vi "TCS_VISA.vi"() -> ()   [LabVIEW 2018]
uses:
  RxTx/RxTx.lvclass
  Serial Communication/Serial Communication.lvclass
  Serial Communication/Serial Communication.lvclass/Serial Communication.ctl
panel:
  in  "RxTx.lvclass 2":refnum<class "RxTx.lvclass">
  in  "Serial Communication in":refnum<class "Serial Communication.lvclass">
  in  "RxTx.lvclass":refnum<class "RxTx.lvclass">
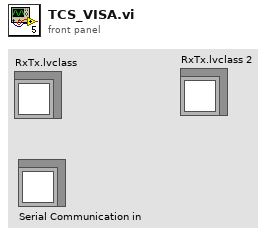
[diagram p1: front panel]
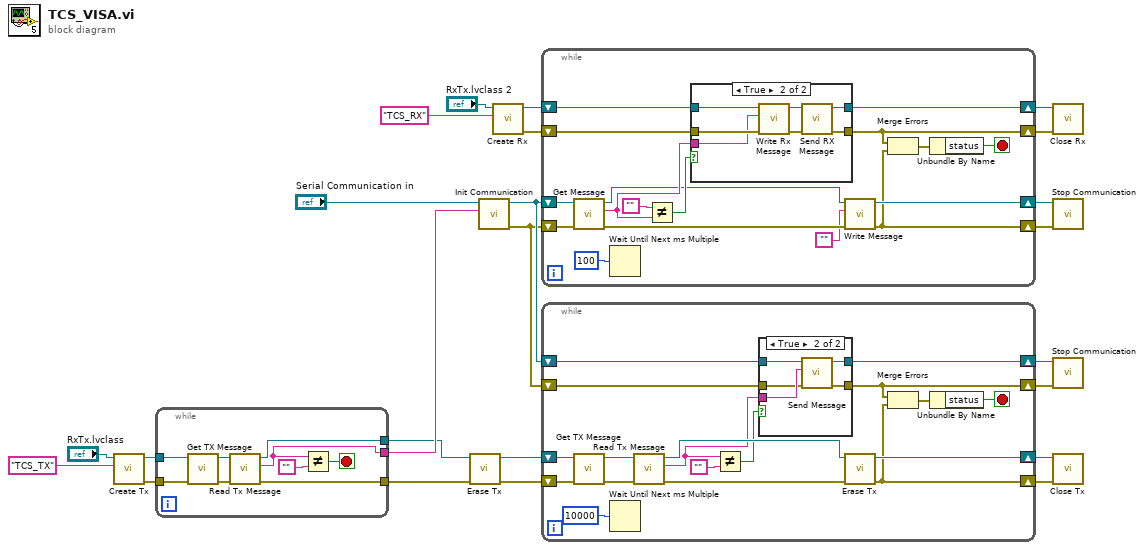
[diagram p0: block diagram]
diagram:
  n1 = call "Create Tx.vi"("Writer Name"="TCS_TX" ("Reader Name"), "RxTx in"="RxTx.lvclass") -> ("error out"=w8:errorcluster, "RxTx out"=w9:refnum<class "RxTx.lvclass">)  [unwired: 8 in]
  n2 = while {
    tunnel: w9 -> [w30]
    tunnel: w8 -> [w29]
    tunnel: [w28] -> w2
    tunnel: [w27] -> w1
    tunnel: [w25] -> w7
    stop <- w26 stop-if-true
    n3 = call "Get TX Message.vi"("error in (no error)"=w29, "RxTx in"=w30) -> ("error out"=w33:errorcluster, "RxTx out"=w32:refnum<class "RxTx.lvclass">)  [unwired: 8 in]
    n4 = call "Read Tx Message.vi"("error in (no error)"=w33, "RxTx in"=w32) -> ("error out"=w28:errorcluster, "Tx Message"=w25:string, "RxTx out"=w27:refnum<class "RxTx.lvclass">)  [unwired: 7 in]
    n5 = Not Equal?(x=w25, y="") -> (x != y?=w26:bool)
  }
  n6 = call "Erase Tx.vi"("error in (no error)"=w2, "RxTx in"=w1) -> ("error out"=w4:errorcluster, "RxTx out"=w3:refnum<class "RxTx.lvclass">)  [unwired: 8 in]
  n7 = call "Init Communication.vi"("VISA resource name"=w7, "Serial Communication in"="Serial Communication in") -> ("error out"=w5:errorcluster, "Serial Communication out"=w6:refnum<class "Serial Communication.lvclass">)  [unwired: 8 in]
  n8 = call "Create Rx.vi"("Reader Name"="TCS_RX", "RxTx in"="RxTx.lvclass 2") -> ("error out"=w14:errorcluster, "RxTx out"=w15:refnum<class "RxTx.lvclass">)  [unwired: 8 in]
  n9 = while {
    shift-right: [w36] -> w10
    shift-left: w5 -> [w43]
    shift-right: [w37] -> w11
    shift-left: w6 -> [w42]
    shift-right: [w46] -> w12
    shift-left: w14 -> [w50]
    shift-right: [w48] -> w13
    shift-left: w15 -> [w49]
    stop <- w34 stop-if-true
    n10 = call "Get Message.vi"("error in (no error)"=w43, "Serial Communication in"=w42) -> ("error out"=w39:errorcluster, "Message"=w41:string, "Serial Communication out"=w40:refnum<class "Serial Communication.lvclass">)  [unwired: 7 in]
    n11 = Wait Until Next ms Multiple(millisecond multiple=u32 100 ("milliseconds to wait")) -> ()  [unwired: 1 out]
    n12 = Not Equal?(x="", y=w41) -> (x != y?=w44:bool)
    n13 = case shown="True" w44 {
      tunnel: w50 -> [w51 w57]
      tunnel: w49 -> [w52 w56]
      tunnel: w41 -> [_ w55]
      tunnel: [w52 w54] -> w48
      tunnel: [w51 w53] -> w46
      frame False {
      }
      frame True {
        n14 = call "Write Rx Message.vi"("error in (no error)"=w57, "Rx Message"=w55, "RxTx in"=w56) -> ("error out"=w58:errorcluster, "RxTx out"=w59:refnum<class "RxTx.lvclass">)  [unwired: 7 in]
        n15 = call "Send RX Message.vi"("error in (no error)"=w58, "RxTx in"=w59) -> ("error out"=w53:errorcluster, "RxTx out"=w54:refnum<class "RxTx.lvclass">)  [unwired: 8 in]
      }
    }
    n16 = call "Write Message.vi"("error in (no error)"=w39, "Message"="", "Serial Communication in"=w40) -> ("error out"=w36:errorcluster, "Serial Communication out"=w37:refnum<class "Serial Communication.lvclass">)  [unwired: 7 in]
    n17 = Merge Errors(w46, w36) -> (w47:errorcluster)
    n18 = Unbundle By Name(w47) -> ("status"=w34:bool)
  }
  n19 = while {
    shift-right: [w69] -> w19
    shift-left: w5 -> [w71]
    shift-right: [w70] -> w20
    shift-left: w6 -> [w72]
    shift-right: [w64] -> w22
    shift-left: w4 -> [w73]
    shift-right: [w66] -> w23
    shift-left: w3 -> [w74]
    stop <- w60 stop-if-true
    n20 = call "Get TX Message.vi"("error in (no error)"=w73, "RxTx in"=w74) -> ("error out"=w76:errorcluster, "RxTx out"=w75:refnum<class "RxTx.lvclass">)  [unwired: 8 in]
    n21 = Wait Until Next ms Multiple(millisecond multiple=u32 10000 ("milliseconds to wait")) -> ()  [unwired: 1 out]
    n22 = call "Read Tx Message.vi"("error in (no error)"=w76, "RxTx in"=w75) -> ("error out"=w65:errorcluster, "Tx Message"=w61:string, "RxTx out"=w67:refnum<class "RxTx.lvclass">)  [unwired: 7 in]
    n23 = Not Equal?(x=w61, y="") -> (x != y?=w63:bool)
    n24 = case shown="True" w63 {
      tunnel: w72 -> [w79 w80]
      tunnel: w71 -> [w78 w83]
      tunnel: [w79 w81] -> w70
      tunnel: w61 -> [_ w84]
      tunnel: [w78 w82] -> w69
      frame False {
      }
      frame True {
        n25 = call "Send Message.vi"("error in (no error)"=w83, "Message"=w84, "Serial Communication in"=w80) -> ("error out"=w82:errorcluster, "Serial Communication out"=w81:refnum<class "Serial Communication.lvclass">)  [unwired: 7 in]
      }
    }
    n26 = call "Erase Tx.vi"("error in (no error)"=w65, "RxTx in"=w67) -> ("error out"=w64:errorcluster, "RxTx out"=w66:refnum<class "RxTx.lvclass">)  [unwired: 8 in]
    n27 = Merge Errors(w69, w64) -> (w77:errorcluster)
    n28 = Unbundle By Name(w77) -> ("status"=w60:bool)
  }
  n29 = call "Close Rx.vi"("error in (no error)"=w12, "RxTx in"=w13) -> ()  [unwired: 8 in, 2 out]
  n30 = call "Stop Communication.vi"("error in (no error)"=w10, "Serial Communication in"=w11) -> ()  [unwired: 8 in, 2 out]
  n31 = call "Stop Communication.vi"("error in (no error)"=w19, "Serial Communication in"=w20) -> ()  [unwired: 8 in, 2 out]
  n32 = call "Close Tx.vi"("error in (no error)"=w22, "RxTx in"=w23) -> ()  [unwired: 8 in, 2 out]
